vi "DAQ_For_Spectrometer.vi"(9 "Condition (>condition Fire )":dbl, 10 "Period (Sec)":dbl=140.0 format="%#_13g", 11 "milliseconds to wait":u32=1000) -> ()   [LabVIEW 2020]
uses:
  <vilib>/Utility/error.llb/DialogType.ctl
  <vilib>/DAQmx/write.llb/DAQmx Write (Digital Bool 1Line 1Point).vi
  <vilib>/DAQmx/read.llb/DAQmx Read (Analog DBL 1Chan 1Samp).vi
  <vilib>/DAQmx/create/channels.llb/DAQmx Create Channel (AI-Voltage-Basic).vi
  <vilib>/DAQmx/configure/timing.llb/DAQmx Timing (Sample Clock).vi
  <vilib>/DAQmx/configure/task.llb/DAQmx Configure Logging (TDMS).vi
  <vilib>/DAQmx/configure/trigger.llb/DAQmx Start Trigger (Digital Edge).vi
  <vilib>/DAQmx/configure/trigger.llb/DAQmx Start Trigger (Time).vi
  <vilib>/DAQmx/configure/trigger.llb/DAQmx Start Trigger (Analog Edge).vi
  <vilib>/DAQmx/miscellaneous.llb/DAQmx Fill In Error Info.vi
  <vilib>/DAQmx/create/channels.llb/DAQmx Create Channel (DO-Digital Output).vi
  <resource>/objmgr/daqmx.rc
panel:
  out "Trigger":bool
  in  "Stop":bool
  out "data":dbl=0.014239551150240004 format="%0.2f"
  in  "Trigger Type":T1(tab)
  in  "Digital Start Trigger Edge":i32(ring)=10280 caption="Edge" items=["Rising"=10280, "Falling"=10171]
  in  "Digital Start Trigger Source":tag="/Dev1/PFI0" caption="Source"
  in  "Digital Pause Trigger Pause When":i32(ring)=10192 caption="Pause When" items=["High"=10192, "Low"=10214]
  in  "Digital Pause Trigger Source":tag="/Dev1/PFI0" caption="Source"
  in  "Analog Start Trigger Level":dbl caption="Level" format="%0.2f"
  in  "Analog Start Trigger Hysteresis":dbl caption="Hysteresis" format="%.2f"
  in  "Analog Start Trigger Slope":i32(ring)=10280 caption="Slope" items=["Rising"=10280, "Falling"=10171]
  in  "Analog Start Trigger Source":string="APFI0" caption="Source"
  in  "Analog Pause Trigger Source":string="APFI0" caption="Source"
  in  "Analog Pause Trigger Pause When":i32(ring)=10093 caption="Pause When" items=["Above Level"=10093, "Below Level"=10107]
  in  "Analog Pause Trigger Level":dbl caption="Level" format="%.2f"
  in  "When":timestamp
  in  "Select Time\nManually":bool
  in  "Number of Samples":i32=1
  in  "TDMS File Path":path
  in  "Sample Rate":dbl=1.0
  in  "Sample Clock Source":tag="OnboardClock"
  in  "Terminal Configuration":i32(ring)=-1 items=["default"=-1, "RSE"=10083, "NRSE"=10078, "Differential"=10106, "Pseudodifferential"=12529]
  in  "Max Voltage":dbl=5.0
  in  "Min Voltage":dbl=-5.0
  in  "Physical Channel":tag="myDAQ1/ai0"
  out "Actual Sample Rate":dbl=1.0 format="%0.2f"
  in  "Logging Mode":i32(ring)=10231 items=["Off"=10231, "Log and Read"=15842]
  in  "Stop Index":dbl=100.0
  in  "stop":bool
  out "PulseNumber Now":dbl=50.0
  out "Pulse Number":dbl=50.0
  out "Waveform Chart":i32(graph)
  out "floor(x/y) 2":i32
  out "floor(x/y)":dbl=139.0
  out "TTL ?":bool=TRUE
  out "Time Index":i32=139
  # "To enable triggers, select a tab above, and configure the settings.\n\nNot all hardware supports all trigger types. Refer to your device documentation for more information."
  # "This trigger type is not supported in continuous sample timing. \n\nRefer to your device documentation for more information on which triggers are supported."
  # "This trigger type is not supported in continuous sample timing. \n\nRefer to your device documentation for more information on which triggers are supported."
  # "If time is not manually set, task will begin after 10 seconds"
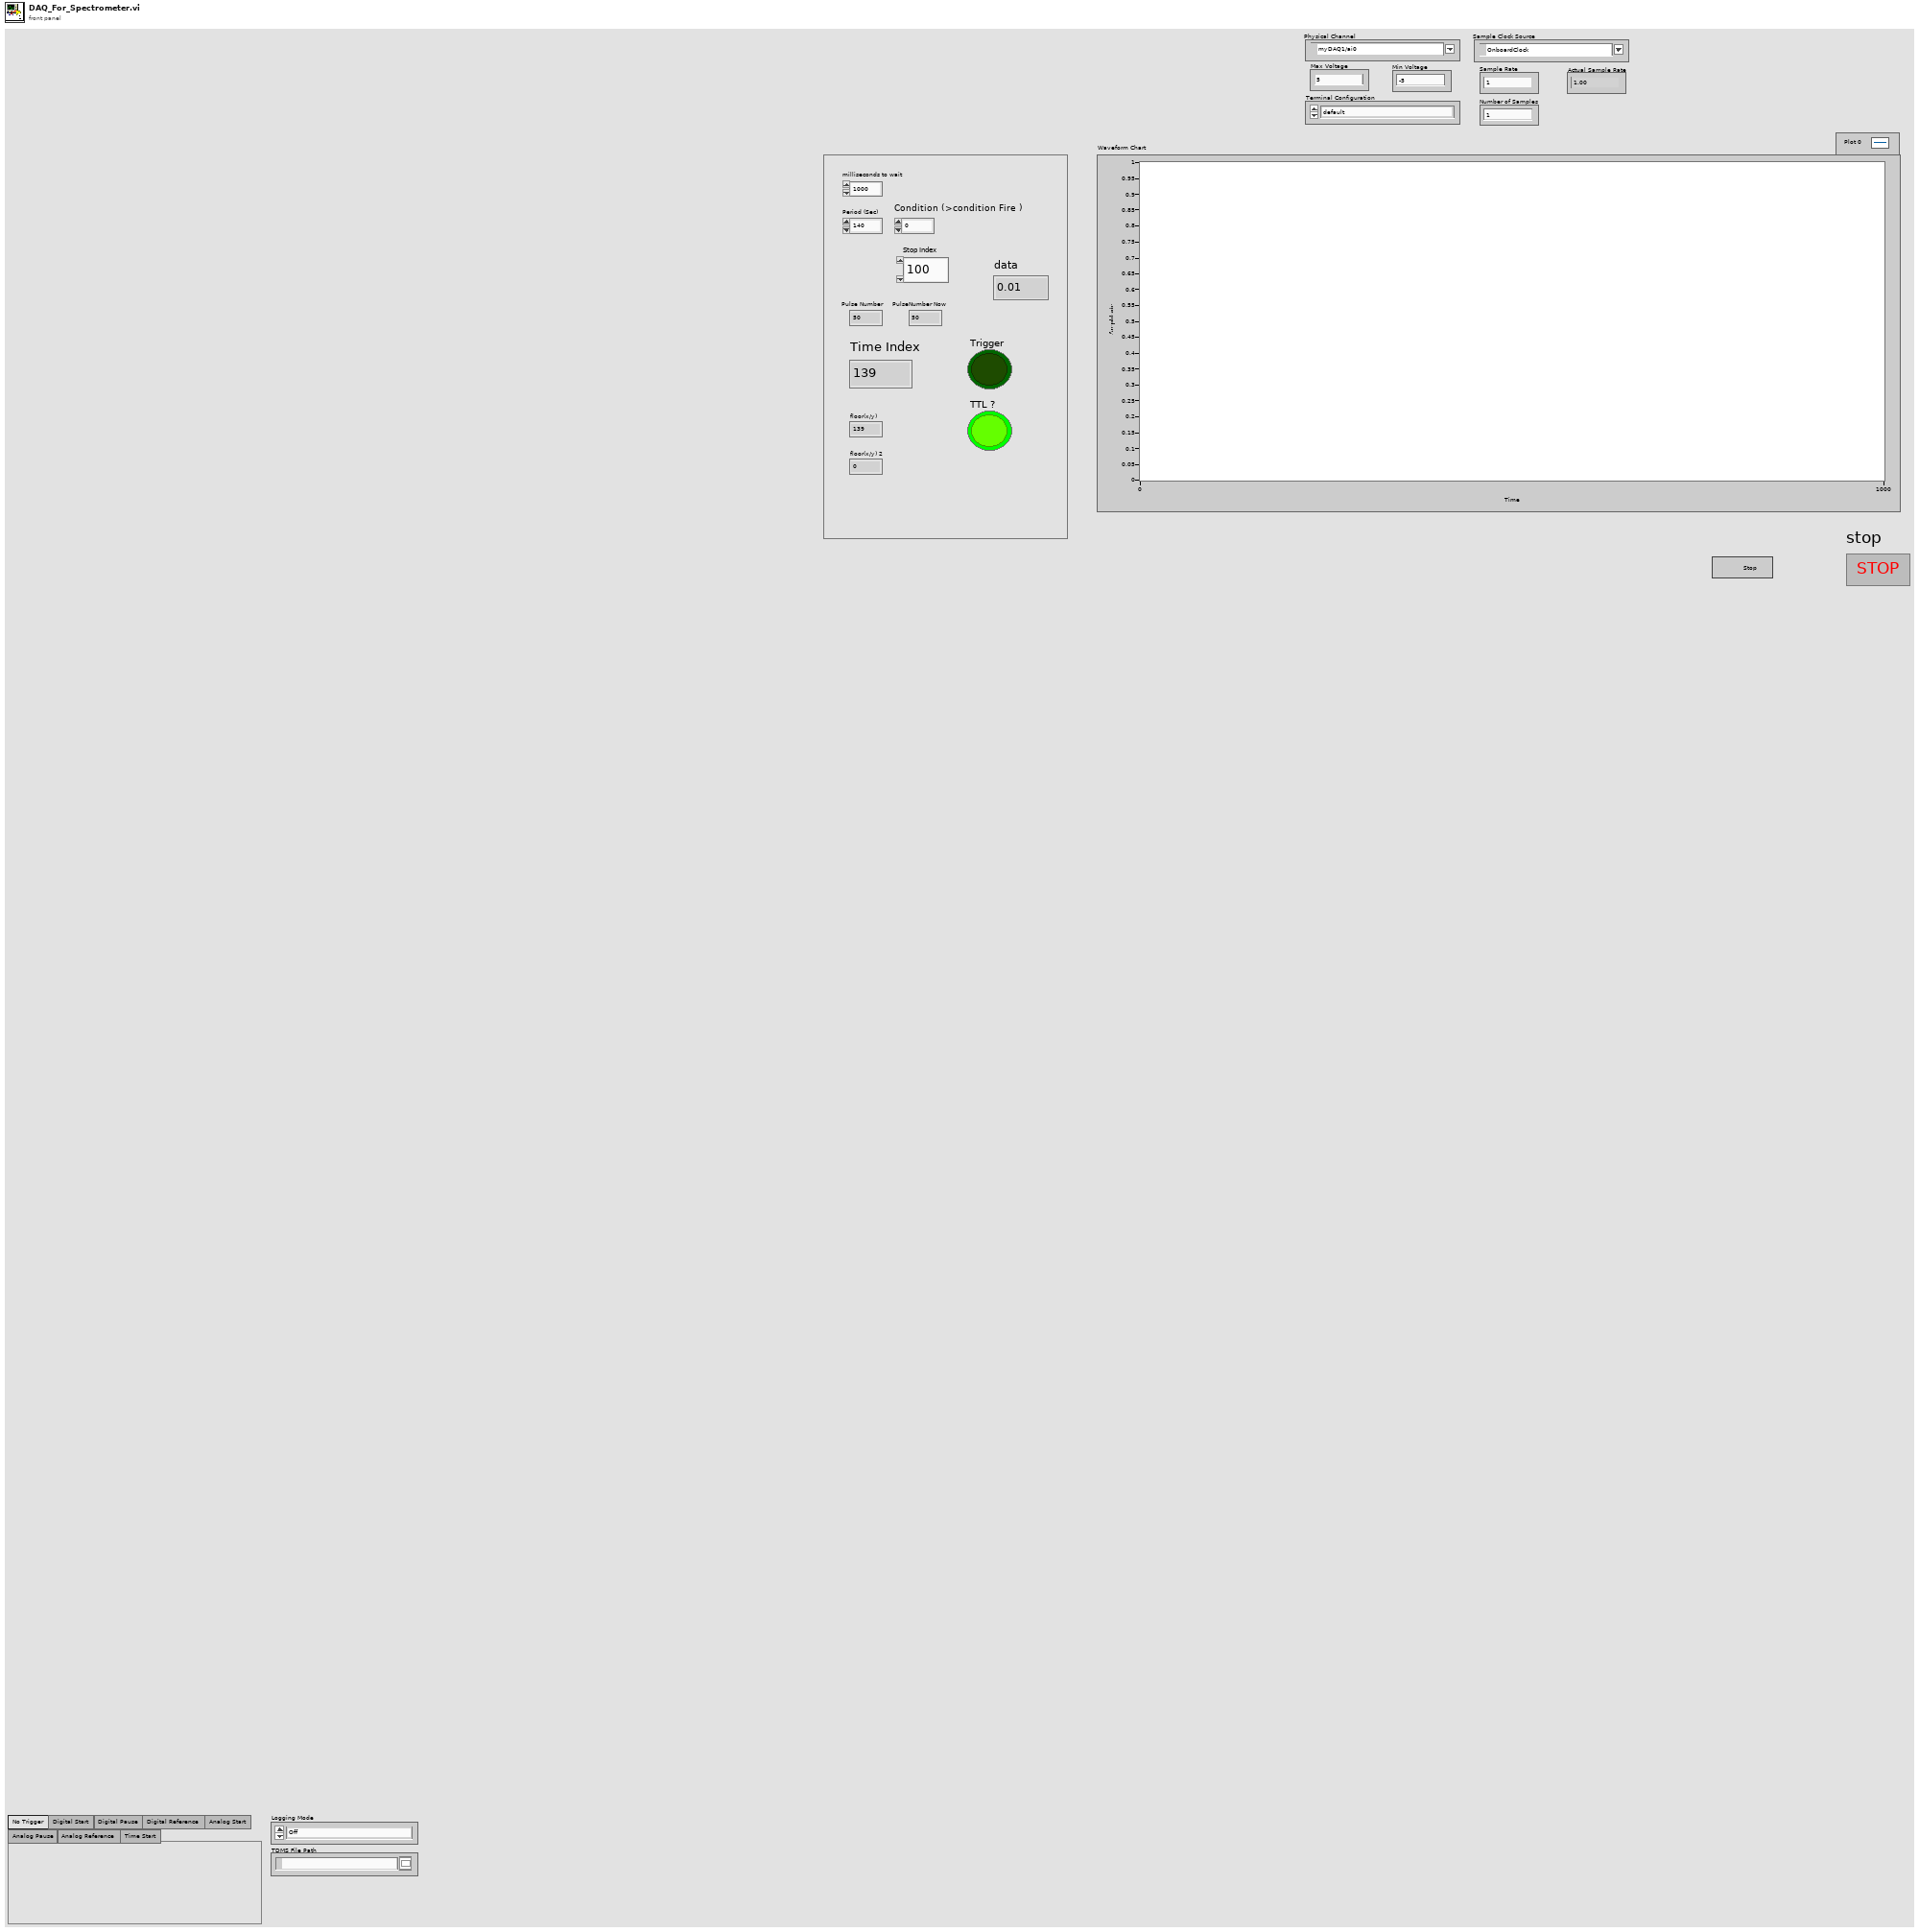
[diagram p1: front panel]
types:
  T1 = enum32{"No Trigger", "Digital Start", "Digital Pause", "Digital Reference", "Analog Start", "Analog Pause", "Analog Reference", "Time Start"}
  T2 = typedef "DialogType.ctl" = u16
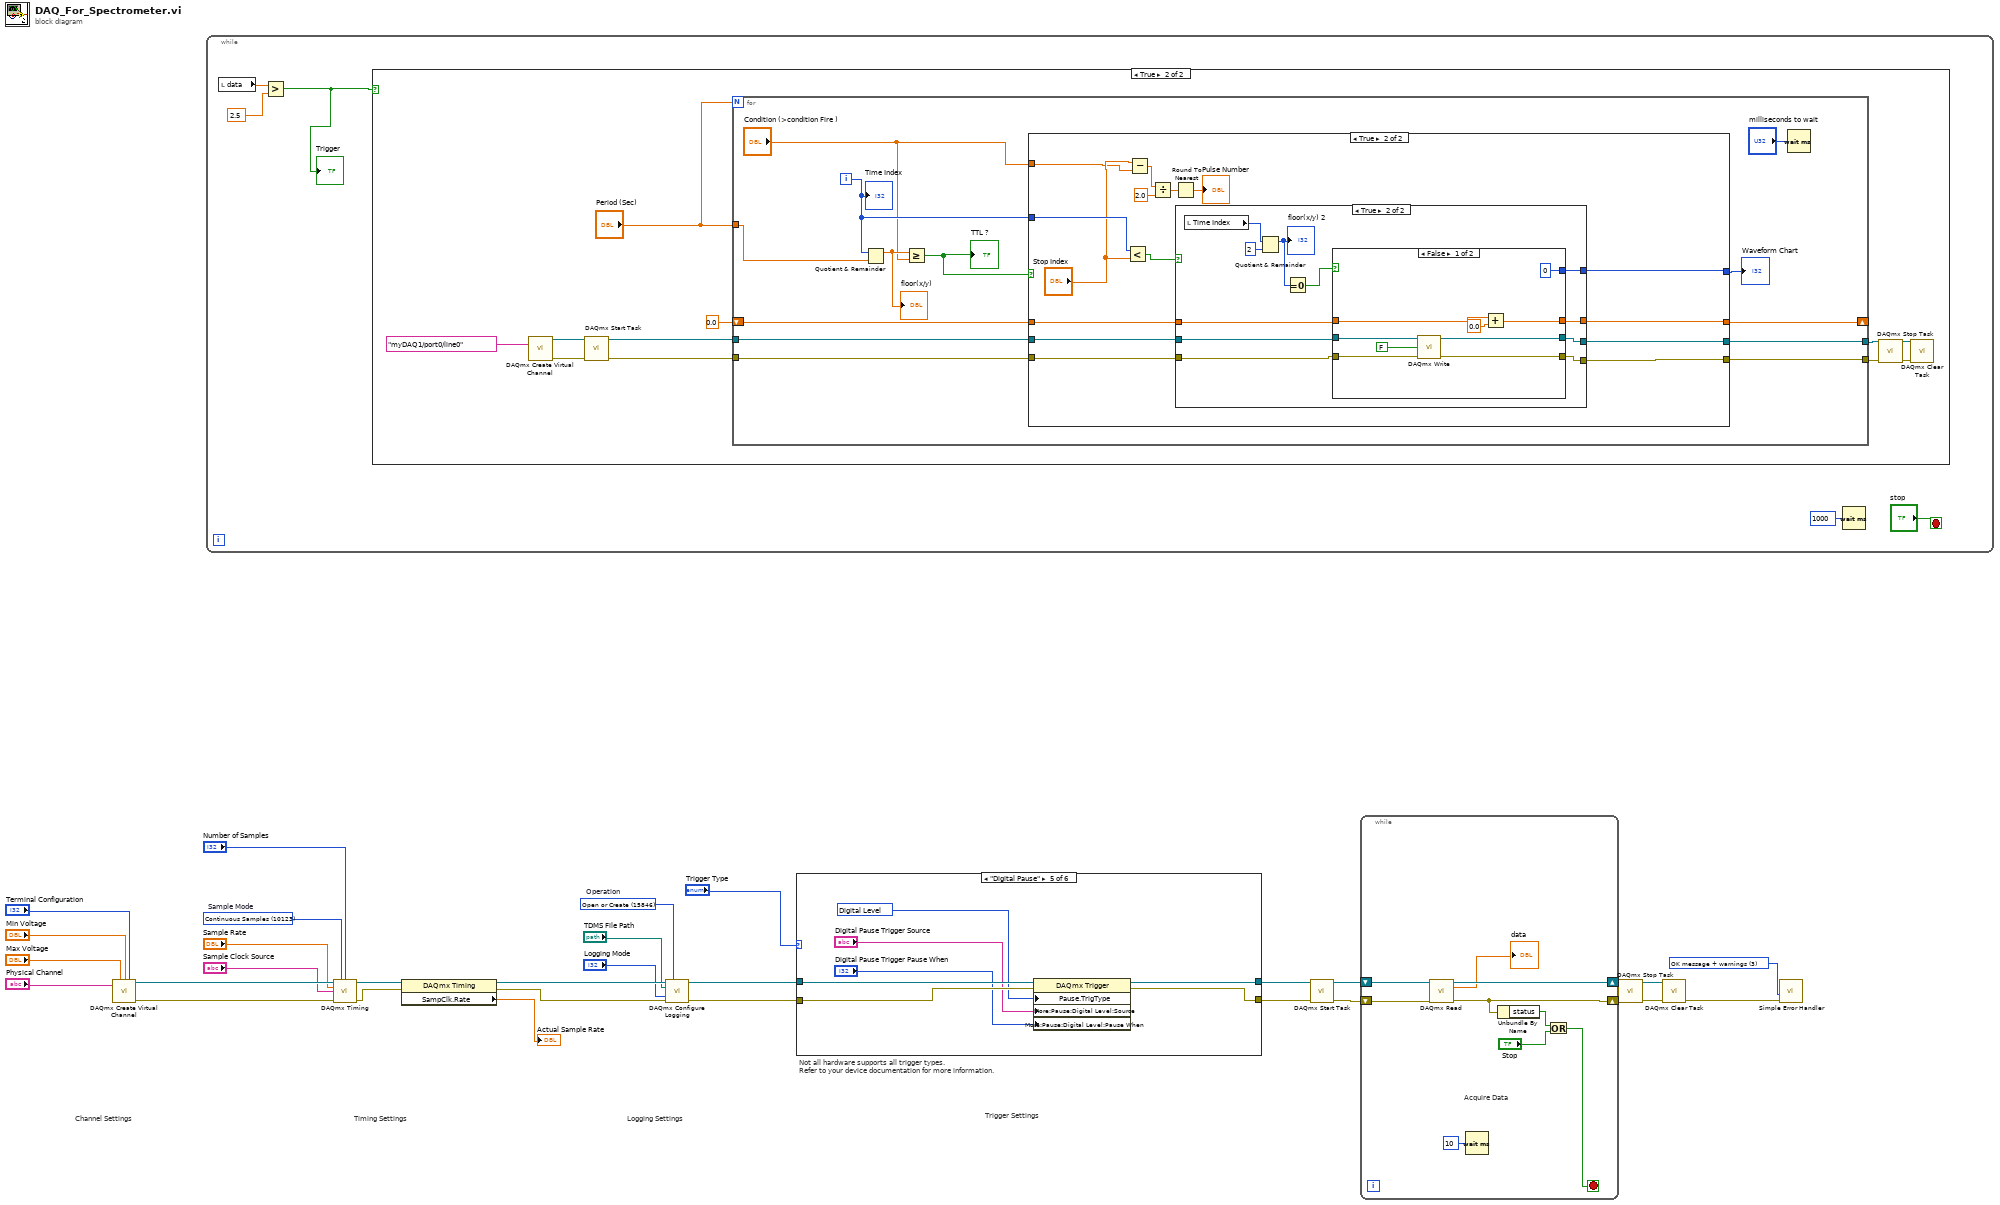
[diagram p0: block diagram]
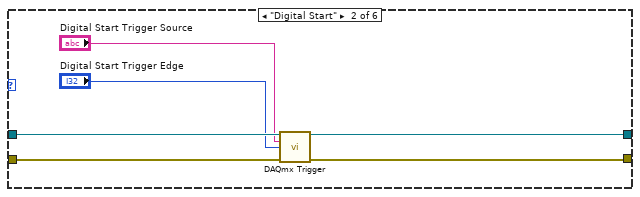
[diagram p3: hidden frame]
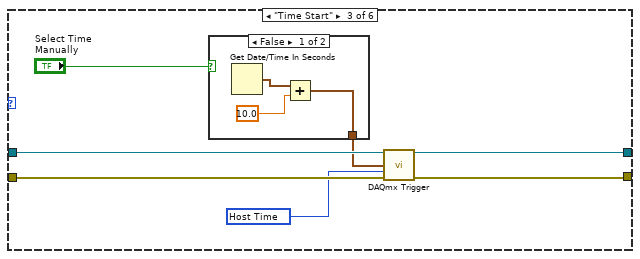
[diagram p4: hidden frame]
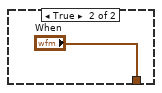
[diagram p5: hidden frame]
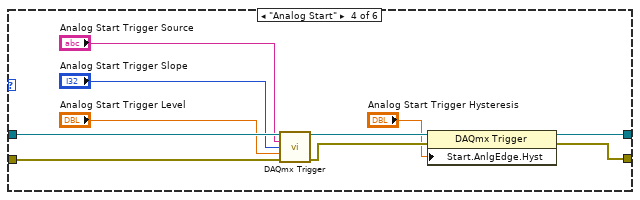
[diagram p6: hidden frame]
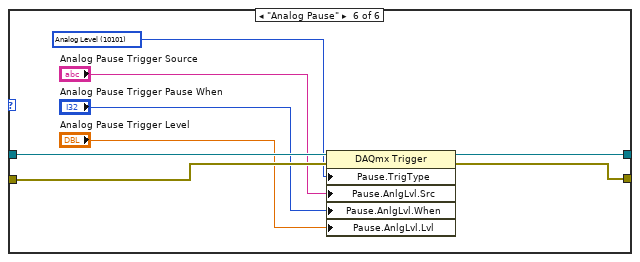
[diagram p7: hidden frame]
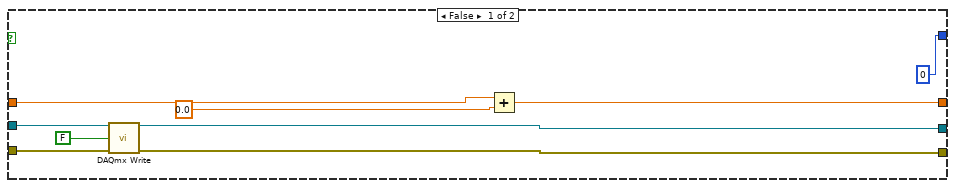
[diagram p9: hidden frame]
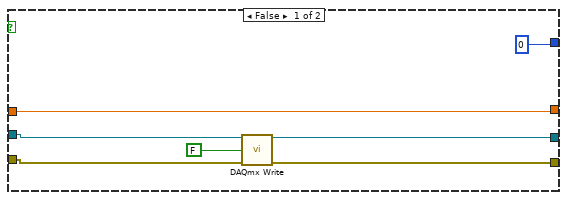
[diagram p10: hidden frame]
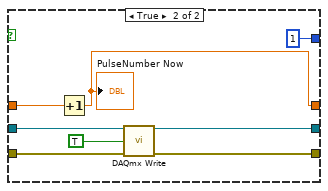
[diagram p11: hidden frame]
diagram:
  w6 = T2 3 items=["no dialog", "OK message", "continue or stop message", "OK message + warnings", "continue/stop + warnings"] ("type of dialog (OK msg:1)")
  w24 = 15846 items=["Open"=10437, "Open or Create"=15846, "Create or Replace"=15847, "Create"=15848]  # Operation
  w29 = 10123 items=["Finite Samples"=10178, "Continuous Samples"=10123, "Hardware Timed Single Point"=12522]  # Sample Mode
  # "Trigger Settings"
  # "Not all hardware supports all trigger types.\nRefer to your device documentation for more information."
  # "Timing Settings"
  # "Channel Settings"
  # "Logging Settings"
  n1 = call-poly <vilib>:"DAQmx Create Virtual Channel.vi"("maximum value"="Max Voltage", "minimum value"="Min Voltage", "input terminal configuration"="Terminal Configuration", "physical channels"="Physical Channel") -> ("task out"=w27:refnum<k21>, "error out"=w28:errorcluster)  [unwired: 10 in]
  n2 = while {
    stop <- "stop" stop-if-true
    n3 = local read "data"() -> (w34:dbl)
    n4 = Greater?(x=w34, y=2.5) -> (0:w32:bool)
    "Trigger" <- w32
    n5 = case shown="True" w32 {
      frame False {
      }
      frame True {
        n6 = call-poly <vilib>:"DAQmx Create Virtual Channel.vi"("lines"=tag "myDAQ1/port0/line0") -> ("task out"=w46:refnum<k21>, "error out"=w45:errorcluster)  [unwired: 13 in]
        n7 = call <vilib>:"DAQmx Start Task.vi"("task/channels in"=w46, "error in"=w45) -> ("task out"=w43:refnum<k21>, "error out"=w42:errorcluster)  [unwired: 12 in]
        n8 = for {
          N: "Period (Sec)" -> [_]
          shift-right: [w49] -> _
          shift-left: 0.0 -> [w56]
          tunnel: w43 -> [w55]
          tunnel: w42 -> [w54]
          tunnel: [w50] -> w39
          tunnel: [w51] -> w38
          tunnel: "Period (Sec)" -> [w53]
          i -> [w52]
          n9 = Quotient & Remainder(x=w52, y=w53) -> (x-y*floor(x/y)=w59:dbl)  [unwired: 1 out]
          "floor(x/y)" <- w59
          n10 = Greater Or Equal?(x=w59, y="Condition (>condition Fire )") -> (x >= y?=w58:bool)
          "TTL ?" <- w58
          n11 = case shown="True" w58 {
            tunnel: [0 w78] -> w57
            tunnel: [w66 w81] -> w49
            tunnel: w56 -> [w67 w84]
            tunnel: w55 -> [w62 w83]
            tunnel: w54 -> [w65 w82]
            tunnel: [w63 w80] -> w50
            tunnel: [w64 w79] -> w51
            tunnel: w52 -> [_ w77]
            tunnel: "Condition (>condition Fire )" -> [_ w70]
            frame False {
              n12 = call-poly <vilib>:"DAQmx Write.vi"("task/channels in"=w62, "data"=FALSE, "error in"=w65) -> ("task out"=w63:refnum<k21>, "error out"=w64:errorcluster)  [unwired: 10 in, 1 out]
              n13 = Add(x=w67, y=0.0) -> (x+y=w66:dbl)
            }
            frame True {
              n14 = Less?(x=w77, y="Stop Index") -> (x < y?=w76:bool)
              n15 = Subtract(x="Stop Index", y=w70) -> (x-y=w73:dbl)
              n16 = Divide(x=w73, y=2.0) -> (x/y=w74:dbl)
              n17 = Round To Nearest(number=w74) -> (nearest integer value=→"Pulse Number":dbl)
              n18 = case shown="True" w76 {
                tunnel: w84 -> [w88 w98]
                tunnel: w83 -> [w90 w97]
                tunnel: w82 -> [w89 w96]
                tunnel: [w88 w95] -> w81
                tunnel: [w85 w94] -> w80
                tunnel: [w86 w93] -> w79
                tunnel: [0 w92] -> w78
                frame False {
                  n19 = call-poly <vilib>:"DAQmx Write.vi"("task/channels in"=w90, "data"=FALSE, "error in"=w89) -> ("task out"=w85:refnum<k21>, "error out"=w86:errorcluster)  [unwired: 10 in, 1 out]
                }
                frame True {
                  n20 = local read "Time Index"() -> (w100:i32)
                  n21 = Quotient & Remainder(x=w100, y=2) -> (x-y*floor(x/y)=w102:i32)  [unwired: 1 out]
                  "floor(x/y) 2" <- w102
                  n22 = Equal To 0?(x=w102) -> (x = 0?=w101:bool)
                  n23 = case shown="False" w101 {
                    tunnel: [0 1] -> w92
                    tunnel: [w108 w118] -> w95
                    tunnel: w98 -> [w110 w117]
                    tunnel: w97 -> [w104 w116]
                    tunnel: w96 -> [w107 w115]
                    tunnel: [w105 w114] -> w94
                    tunnel: [w106 w113] -> w93
                    frame False {
                      n24 = call-poly <vilib>:"DAQmx Write.vi"("task/channels in"=w104, "data"=FALSE, "error in"=w107) -> ("task out"=w105:refnum<k21>, "error out"=w106:errorcluster)  [unwired: 10 in, 1 out]
                      n25 = Add(x=w110, y=0.0) -> (x+y=w108:dbl)
                    }
                    frame True {
                      n26 = Increment(x=w117) -> (x+1=w118:dbl)
                      "PulseNumber Now" <- w118
                      n27 = call-poly <vilib>:"DAQmx Write.vi"("task/channels in"=w116, "data"=TRUE, "error in"=w115) -> ("task out"=w114:refnum<k21>, "error out"=w113:errorcluster)  [unwired: 10 in, 1 out]
                    }
                  }
                }
              }
            }
          }
          "Waveform Chart" <- w57
          n28 = Wait (ms)(milliseconds to wait="milliseconds to wait") -> ()  [unwired: 1 out]
          "Time Index" <- w52
        }
        n29 = call <vilib>:"DAQmx Stop Task.vi"("task/channels in"=w39, "error in"=w38) -> ("task out"=w41:refnum<k21>, "error out"=w40:errorcluster)  [unwired: 12 in]
        n30 = call <vilib>:"DAQmx Clear Task.vi"("task in"=w41, "error in"=w40) -> ()  [unwired: 13 in, 1 out]
      }
    }
    n31 = Wait (ms)(milliseconds to wait=u32 1000) -> ()  [unwired: 1 out]
  }
  n32 = call-poly <vilib>:"DAQmx Timing.vi"("task/channels in"=w27, "sample mode"=w29, "samples per channel"="Number of Samples", "rate"="Sample Rate", "source"="Sample Clock Source", "error in"=w28) -> ("task out"=w31:refnum<k21>, "error out"=w30:errorcluster)  [unwired: 8 in]
  n33 = property class="DAQmx Timing"(reference=w31, error in=w30) -> (reference out=w26:refnum<k21>, error out=w25:errorcluster, "SampClk.Rate"=→"Actual Sample Rate":dbl)
  n34 = call-poly <vilib>:"DAQmx Configure Logging.vi"("task/channels in"=w26, "operation"=w24, "file path"="TDMS File Path", "logging mode"="Logging Mode", "error in"=w25) -> ("task out"=w4:refnum<k21>, "error out"=w3:errorcluster)  [unwired: 9 in]
  n35 = case shown="\"Digital Pause\"" "Trigger Type" {
    tunnel: w4 -> [w121 w127 w134 w148 w155 w163]
    tunnel: w3 -> [w120 w126 w133 w147 w152 w160]
    tunnel: [w121 w125 w132 w145 w154 w162] -> w1
    tunnel: [w120 w124 w131 w144 w153 w161] -> w2
    frame "No Trigger", Default {
    }
    frame "Digital Start" {
      n36 = call-poly <vilib>:"DAQmx Trigger.vi"("task/channels in"=w127, "source"="Digital Start Trigger Source", "edge"="Digital Start Trigger Edge", "error in"=w126) -> ("task out"=w125:refnum<k21>, "error out"=w124:errorcluster)  [unwired: 10 in]
    }
    frame "Time Start" {
      w130 = 16126 items=["Host Time"=16126, "I/O Device Time"=16127] ("timescale")
      n37 = case shown="False" "Select Time\nManually" {
        tunnel: [w135 "When"] -> w128
        frame False {
          n38 = Get Date/Time In Seconds() -> (seconds since 1Jan1904=w137:timestamp)
          n39 = Add(x=w137, y=10.0) -> (x+y=w135:timestamp)
        }
        frame True {
        }
      }
      n40 = call-poly <vilib>:"DAQmx Trigger.vi"("task/channels in"=w134, "when"=w128, "timescale"=w130, "error in"=w133) -> ("task out"=w132:refnum<k21>, "error out"=w131:errorcluster)  [unwired: 10 in]
    }
    frame "Analog Start" {
      n41 = call-poly <vilib>:"DAQmx Trigger.vi"("task/channels in"=w148, "source"="Analog Start Trigger Source", "slope"="Analog Start Trigger Slope", "level"="Analog Start Trigger Level", "error in"=w147) -> ("task out"=w143:refnum<k21>, "error out"=w142:errorcluster)  [unwired: 9 in]
      n42 = property class="DAQmx Trigger"(reference=w143, error in=w142, "Start.AnlgEdge.Hyst"="Analog Start Trigger Hysteresis") -> (reference out=w145:refnum<k21>, error out=w144:errorcluster)
    }
    frame "Digital Pause" {
      w151 = 10152 items=["Analog Level"=10101, "Analog Window"=10103, "Digital Level"=10152, "Digital Pattern"=10398, "None"=10230] ("Pause.TrigType")
      n43 = property class="DAQmx Trigger"(reference=w155, error in=w152, "Pause.TrigType"=w151, "More:Pause:Digital Level:Source"="Digital Pause Trigger Source", "More:Pause:Digital Level:Pause When"="Digital Pause Trigger Pause When") -> (reference out=w154:refnum<k21>, error out=w153:errorcluster)
    }
    frame "Analog Pause" {
      w159 = 10101 items=["Analog Level"=10101, "Analog Window"=10103, "Digital Level"=10152, "Digital Pattern"=10398, "None"=10230] ("Pause.TrigType")
      n44 = property class="DAQmx Trigger"(reference=w163, error in=w160, "Pause.TrigType"=w159, "Pause.AnlgLvl.Src"="Analog Pause Trigger Source", "Pause.AnlgLvl.When"="Analog Pause Trigger Pause When", "Pause.AnlgLvl.Lvl"="Analog Pause Trigger Level") -> (reference out=w162:refnum<k21>, error out=w161:errorcluster)
    }
  }
  n45 = call <vilib>:"DAQmx Start Task.vi"("task/channels in"=w1, "error in"=w2) -> ("task out"=w23:refnum<k21>, "error out"=w22:errorcluster)  [unwired: 12 in]
  n46 = while {
    shift-right: [w170] -> w10
    shift-left: w23 -> [w172]
    shift-right: [w169] -> w9
    shift-left: w22 -> [w171]
    stop <- w164 stop-if-true
    # "Acquire Data"
    n47 = call-poly <vilib>:"DAQmx Read.vi"("task/channels in"=w172, "error in"=w171) -> ("task out"=w170:refnum<k21>, "data"=→"data":dbl, "error out"=w169:errorcluster)  [unwired: 11 in]
    n48 = Wait (ms)(milliseconds to wait=u32 10) -> ()  [unwired: 1 out]
    n49 = Unbundle By Name(w169) -> ("status"=w167:bool)
    n50 = Or(x=w167, y="Stop") -> (x .or. y?=w164:bool)
  }
  n51 = call <vilib>:"DAQmx Stop Task.vi"("task/channels in"=w10, "error in"=w9) -> ("task out"=w7:refnum<k21>, "error out"=w8:errorcluster)  [unwired: 12 in]
  n52 = call <vilib>:"DAQmx Clear Task.vi"("task in"=w7, "error in"=w8) -> ("error out"=w21:errorcluster)  [unwired: 13 in]
  n53 = call <vilib>:"Simple Error Handler.vi"("type of dialog (OK msg:1)"=w6, "error in (no error)"=w21) -> ()  [unwired: 3 in, 5 out]
